vi "7_读取条形码.vi"() -> ()   [LabVIEW 2020]
uses:
  <vilib>/vision/driver/NI_Vision_Acquisition_Software.lvlib
  <vilib>/vision/NI_Vision_Development_Module.lvlib
panel:
  out "Image":T1(plugin-control)
  in  "Session In":refnum<k21>
  out "error out":errorcluster
  out "Data":string
  in  "停止":bool
  in  "Image Type":T2 items=["Grayscale (U8)", "Grayscale (I16)", "Grayscale (SGL)", "Complex (CSG)", "RGB (U32)", "HSL (U32)", "RGB (U64)", "Grayscale (U16)"]
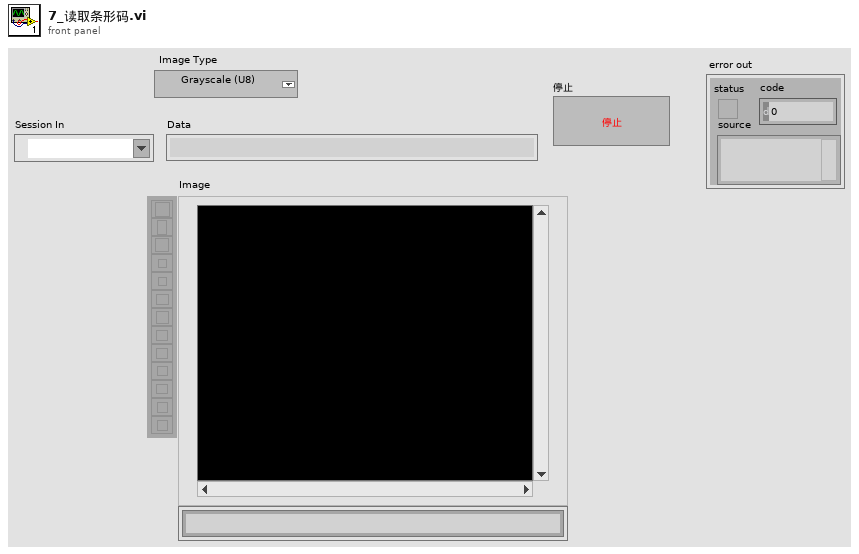
[diagram p1: front panel]
types:
  T1 = typedef "IMAQ Image.ctl" = refnum<image>
  T2 = typedef "Image Type" = u32
  T3 = cluster{"Data":string, "Special Char 1":string, "Special Char 2":string, "Checksum(s)":string, "Barcode Type":u32, "Confidence Level":sgl, "Bounding Box":cluster{"x":sgl, "y":sgl}[]}[]
  T4 = cluster{"Data":string, "Special Char 1":string, "Special Char 2":string, "Checksum(s)":string, "Barcode Type":u32, "Confidence Level":sgl, "Bounding Box":cluster{"x":sgl, "y":sgl}[]}
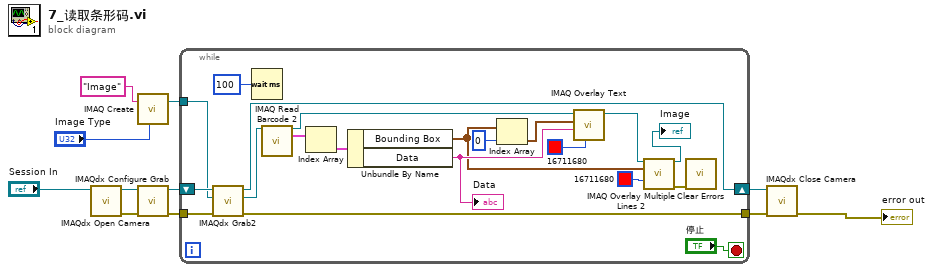
[diagram p0: block diagram]
diagram:
  n1 = call <vilib>:"IMAQdx Open Camera.vi"("Session In"="Session In") -> ("error out"=w10:errorcluster, "Session Out"=w11:refnum<k21>)  [unwired: 9 in]
  n2 = call "IMAQ Create"("Image Name"="Image", "Image Type"="Image Type") -> ("New Image"=w7:T1)  [unwired: 3 in, 1 out]
  n3 = call <vilib>:"IMAQdx Configure Grab.vi"("error in"=w10, "Session In"=w11) -> ("error out"=w9:errorcluster, "Session Out"=w8:refnum<k21>)  [unwired: 8 in]
  n4 = while {
    tunnel: w9 -> [w31]
    tunnel: w7 -> [w29]
    shift-right: [w27] -> w4
    shift-left: w8 -> [w30]
    tunnel: [w22] -> w3
    stop <- "停止" stop-if-true
    n5 = call <vilib>:"IMAQdx Grab2.vi"("error in"=w31, "Image In"=w29, "Session In"=w30) -> ("error out"=w22:errorcluster, "Image Out"=w25:T1, "Session Out"=w27:refnum<k21>)  [unwired: 5 in, 1 out]
    n6 = Wait (ms)(milliseconds to wait=u32 100 ("等待时间（毫秒）")) -> ()  [unwired: 1 out]
    n7 = call "IMAQ Read Barcode 2"("Image"=w25) -> ("Image (duplicate)"=w21:T1, "Barcodes"=w24:T3)  [unwired: 10 in, 3 out]
    n8 = Index Array(array=w24) -> (element=w23:T4)  [unwired: 1 in]
    n9 = Unbundle By Name(w23) -> ("Bounding Box"=w16:cluster{"x":sgl, "y":sgl}[], "Data"=w18:string)
    "Data" <- w18
    n10 = Index Array(array=w16, index=0 ("索引")) -> (element=w19:cluster{"x":sgl, "y":sgl})
    n11 = call "IMAQ Overlay Text"("Text Color (black)"=u32 16711680, "String"=w18, "Origin"=w19, "Image"=w21) -> ("Image Out"=w12:T1)  [unwired: 6 in, 1 out]
    n12 = call "IMAQ Overlay Multiple Lines 2"("Image"=w12, "Line End Points"=w16, "Color"=u32 16711680) -> ("Image Out"=→"Image":T1, "error out"=w14:errorcluster)  [unwired: 11 in]
    n13 = call <vilib>:"Clear Errors.vi"("error in (no error)"=w14) -> ()  [unwired: 5 in, 2 out]
  }
  n14 = call <vilib>:"IMAQdx Close Camera.vi"("error in"=w3, "Session In"=w4) -> ("error out"=→"error out":errorcluster)  [unwired: 9 in]
